vi "Sample_Scan_Pause_v2.vi"(4 "Z tilt comp":bool, 6 "Microsteps (MS=64)":dbl=64.0, 7 "Tilt x/z":dbl=64.0, 8 "Spacing [microns]":dbl=10.0, 9 "Long Side Speed [micron/s]":dbl=10.0, 10 "Scan Mode":T2 items=["Mode 1", "Mode 2", "Continuous 1", "Continuous 2"], 11 "waypoints path":path=path "C:/Users/ALS Measurement/Google Drive/LabVIEW/Thermionics Manipulator") -> (0 "velocity cluster":T1, 1 "Scan Time (hous:minutes:seconds)":string, 2 "Sample Scan Array":i32[][](array[numeric]), 3 "Problem":bool, 5 "Number of Points":i32)   [LabVIEW 2018]
uses:
  Scan Mode.ctl
  ConversionAndInformation/Unit_Control.ctl
panel:
  out "delta long side M3/1":dbl
  out "delta long side M2":dbl
  out "delta spacing M1/3":dbl
  out "delta spacing M2":dbl
  out "x/y":dbl
  out "in plain angle":dbl
  in  "velocity cluster 2":T1
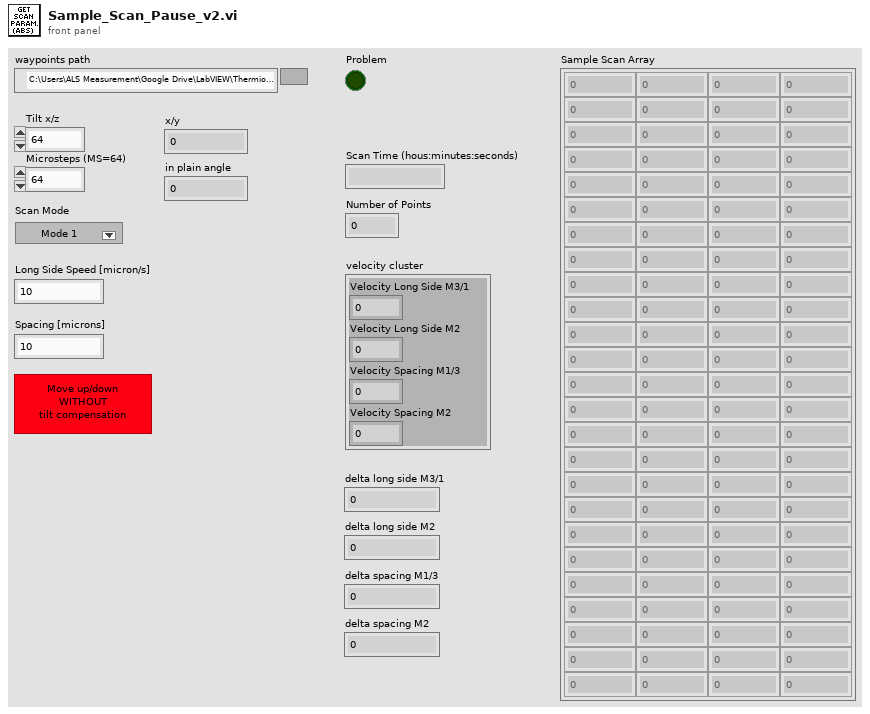
[diagram p1: front panel]
types:
  T1 = cluster{"Velocity Long Side M3/1":dbl, "Velocity Long Side M2":dbl, "Velocity Spacing M1/3":dbl, "Velocity Spacing M2":dbl}
  T2 = typedef "Scan Mode.ctl" = u16
  T3 = typedef "Unit_Control.ctl" = enum16{"Angle (Degrees)", "Rad", "Angle [TMC]", "Microsteps [TMC]", "Inches", "Nanometer", "Meter", "Centimeter", "Millimeter", "Micron"}
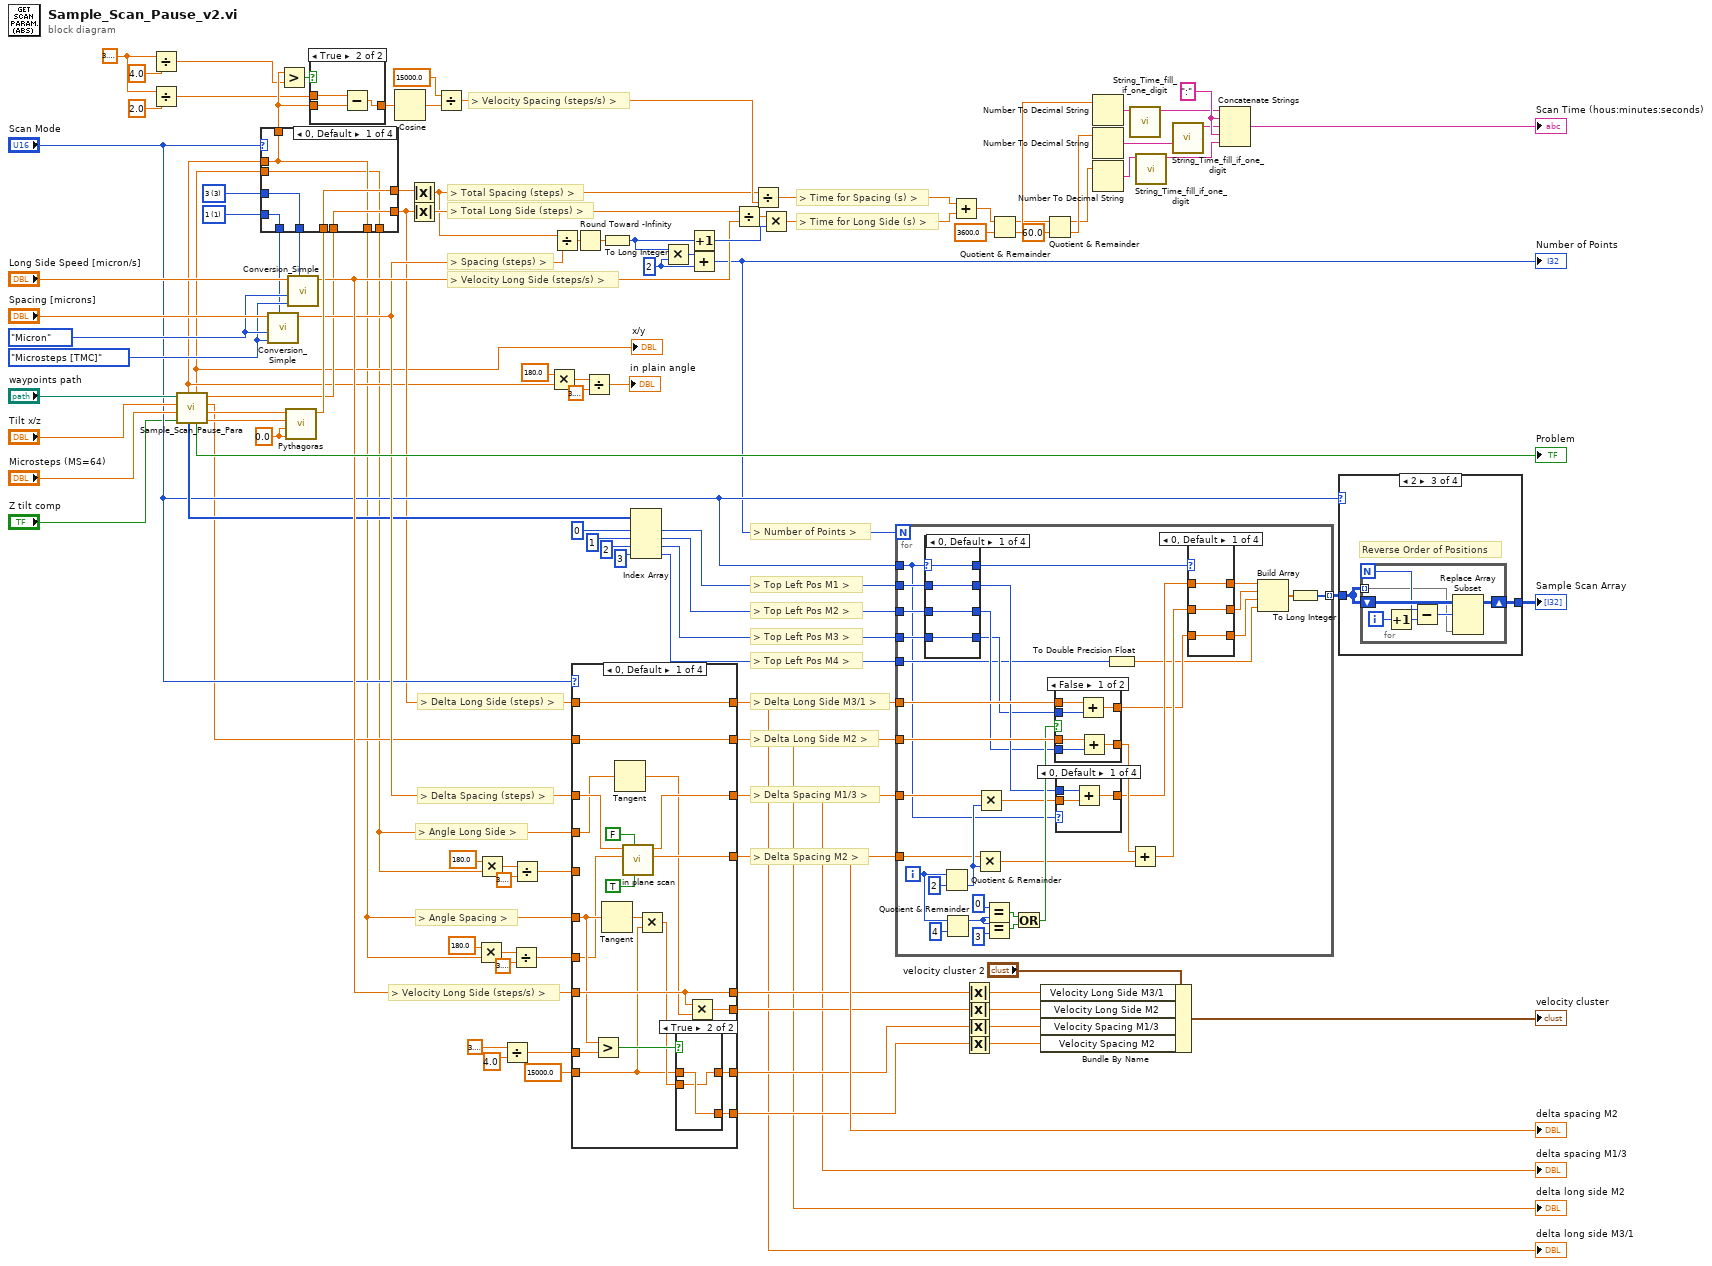
[diagram p0: block diagram]
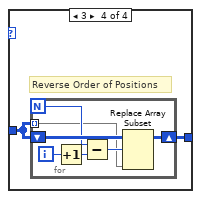
[diagram p4: hidden frame]
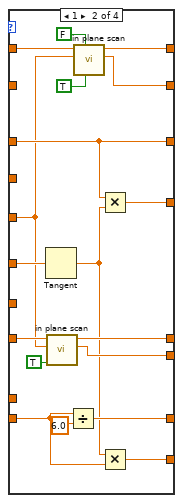
[diagram p6: hidden frame]
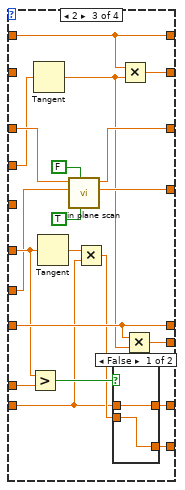
[diagram p7: hidden frame]
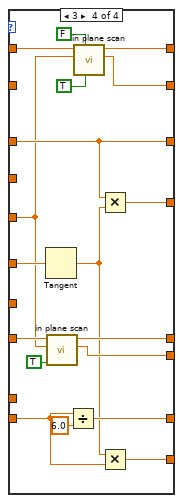
[diagram p9: hidden frame]
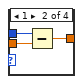
[diagram p10: hidden frame]
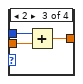
[diagram p11: hidden frame]
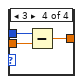
[diagram p12: hidden frame]
diagram:
  w54 = 3.141592653589793
  w79 = u16 3 items=["none", "1", "2", "3", "4", "all"] ("Motor")
  w80 = u16 1 items=["none", "1", "2", "3", "4", "all"] ("Motor")
  w83 = 2 ("y")
  w92 = ":"
  w101 = 0.0 ("Motor 2 Coordinate (bottom right)")
  w66 = Unit_Control."Microsteps [TMC]" ("Output Unit")
  w67 = Unit_Control."Micron" ("Input Unit")
  # "> Velocity Long Side (steps/s) >"
  # "> Top Left Pos M4 >"
  # "> Delta Spacing M2 >"
  # "> Delta Spacing M1/3 >"
  # "> Delta Long Side M2 >"
  # "> Delta Long Side M3/1 >"
  # "> Delta Spacing (steps) >"
  # "> Angle Spacing >"
  # "> Angle Long Side >"
  # "> Number of Points >"
  # "> Delta Long Side (steps) >"
  # "> Top Left Pos M3 >"
  # "> Top Left Pos M2 >"
  # "> Top Left Pos M1 >"
  # "> Time for Long Side (s) >"
  # "> Time for Spacing (s) >"
  # "> Total Long Side (steps) >"
  # "> Total Spacing (steps) >"
  # "> Velocity Spacing (steps/s) >"
  # "> Spacing (steps) >"
  # "> Velocity Long Side (steps/s) >"
  n1 = Divide(x=w54, y=4.0) -> (x/y=w53:dbl)
  n2 = Divide(x=w54, y=2.0) -> (x/y=w52:dbl)
  n3 = call "Sample_Scan_Pause_Para.vi"("Z tilt comp"="Z tilt comp", "Microsteps (MS=64)"="Microsteps (MS=64)", "Tilt x/z"="Tilt x/z", "waypoints path"="waypoints path") -> ("Delta M2 in plain total"=w102:dbl, "Delta M1 in plain total"=w103:dbl, "M2 Z tilt comp total"=w36:dbl, "Delta M3 total"=w35:dbl, "Problem"=→"Problem":bool, "tilt angle (rad)"=w19:dbl, "Top Left Position Array"=w49:i32[], "in plain angle (rad)"=w20:dbl)
  "x/y" <- w19
  n4 = call "Pythagoras.vi"("Motor 2 Coordinate (bottom right)"=w101, "Motor 1 Coordinate (bottom right)"=w101, "Motor 2 Coordinate (top left)"=w102, "Motor 1 Coordinate (top left)"=w103) -> ("In Plain Distance"=w65:dbl)  [unwired: 7 in]
  n5 = case shown="0, Default" "Scan Mode" {
    tunnel: w65 -> [w110 w119 w122 w131]
    tunnel: w35 -> [w113 w116 w125 w128]
    tunnel: [w113 w119 w125 w131] -> w34
    tunnel: [w112 w118 w124 w130] -> w64
    tunnel: [w111 w117 w123 w129] -> w81
    tunnel: w80 -> [w112 w117 w124 w129]
    tunnel: w79 -> [w111 w118 w123 w130]
    tunnel: [w110 w116 w122 w128] -> w5
    tunnel: w20 -> [w109 w114 w121 w126]
    tunnel: w19 -> [w108 w115 w120 w127]
    tunnel: [w109 w115 w121 w127] -> w72
    tunnel: [w109 w115 w121 w127] -> w9
    tunnel: [w108 w114 w120 w126] -> w12
    frame 0, Default {
    }
    frame 1 {
    }
    frame 2 {
    }
    frame 3 {
    }
  }
  n6 = call "Conversion_Simple.vi"("Motor"=w64, "Output Unit"=w66, "Input Unit"=w67, "Input"="Spacing [microns]") -> ("Output"=w57:dbl)  [unwired: 6 in, 1 out]
  n7 = Greater?(x=w72, y=w53) -> (0:w73:bool)
  n8 = call "Conversion_Simple.vi"("Motor"=w81, "Output Unit"=w66, "Input Unit"=w67, "Input"="Long Side Speed [micron/s]") -> ("Output"=w58:dbl)  [unwired: 6 in, 1 out]
  n9 = case shown="True" w73 {
    tunnel: w72 -> [w132 w135]
    tunnel: [w132 w134] -> w51
    tunnel: w52 -> [_ w133]
    frame False {
    }
    frame True {
      n10 = Subtract(x=w133, y=w135) -> (x-y=w134:dbl)
    }
  }
  n11 = Cosine(x=w51) -> (cos(x)=w71:dbl)
  n12 = Absolute Value(x=w5) -> (abs(x)=w4:dbl)
  n13 = Absolute Value(x=w34) -> (abs(x)=w33:dbl)
  n14 = Divide(x=15000.0, y=w71) -> (x/y=w70:dbl)
  n15 = Multiply(x=180.0 ("y"), y=w9) -> (x*y=w10:dbl)
  n16 = Multiply(x=180.0 ("y"), y=w12) -> (x*y=w15:dbl)
  n17 = Divide(x=3.141592653589793, y=4.0) -> (x/y=w38:dbl)
  n18 = Divide(x=w10, y=3.141592653589793) -> (x/y=w6:dbl)
  n19 = Divide(x=w15, y=3.141592653589793) -> (x/y=w7:dbl)
  n20 = Multiply(x=180.0 ("y"), y=w20) -> (x*y=w22:dbl)
  n21 = Divide(x=w4, y=w57) -> (x/y=w100:dbl)
  n22 = case shown="0, Default" "Scan Mode" {
    tunnel: w34 -> [w153 w175 w195 w217]
    tunnel: w9 -> [w140 w161 w181 w203]
    tunnel: w12 -> [w139 _ w180 _]
    tunnel: w57 -> [w152 w172 w194 w214]
    tunnel: [w153 w174 w195 w216] -> w16
    tunnel: [w137 w173 w191 w215] -> w17
    tunnel: [w151 w172 w193 w214] -> w18
    tunnel: [w150 w171 w192 w213] -> w63
    tunnel: w58 -> [w149 w170 w190 w212]
    tunnel: 15000.0 -> [w141 w163 w182 w205]
    tunnel: [w149 w168 w190 w210] -> w32
    tunnel: [w147 w167 w188 w209] -> w30
    tunnel: [w145 w166 w186 w208] -> w28
    tunnel: [w144 w164 w185 w206] -> w26
    tunnel: w38 -> [w138 _ w179 _]
    tunnel: w36 -> [w137 _ _ _]
    tunnel: w7 -> [_ w160 _ w202]
    tunnel: w6 -> [w136 _ w178 _]
    frame 0, Default {
      n23 = Greater?(x=w140, y=w138) -> (0:w146:bool)
      n24 = Tangent(1:w140) -> (0:w142:dbl)
      n25 = Tangent(1:w139) -> (0:w148:dbl)
      n26 = call "in plane scan.vi"("invert y"=TRUE, "invert x"=FALSE, "angle (degrees)"=w136, "v total"=w152) -> ("v_y"=w150:dbl, "v_x"=w151:dbl)  [unwired: 2 in, 4 out]
      n27 = Multiply(x=w142, y=w141) -> (x*y=w143:dbl)
      n28 = case shown="True" w146 {
        tunnel: w141 -> [w157 w159]
        tunnel: [w157 w158] -> w145
        tunnel: [w156 w159] -> w144
        tunnel: w143 -> [w156 w158]
        frame False {
        }
        frame True {
        }
      }
      n29 = Multiply(x=w149, y=w148) -> (x*y=w147:dbl)
    }
    frame 1 {
      n30 = Tangent(1:w161) -> (0:w162:dbl)
      n31 = call "in plane scan.vi"("abs(x,y)"=TRUE ("invert y"), "angle (degrees)"=w160, "v total"=w170) -> ("v_y"=w167:dbl, "v_x"=w168:dbl)  [unwired: 3 in, 4 out]
      n32 = Divide(x=w163, y=6.0) -> (x/y=w166:dbl)
      n33 = call "in plane scan.vi"("invert y"=TRUE, "invert x"=FALSE, "angle (degrees)"=w160, "v total"=w175) -> ("v_y"=w173:dbl, "v_x"=w174:dbl)  [unwired: 2 in, 4 out]
      n34 = Multiply(x=w172, y=w162) -> (x*y=w171:dbl)
      n35 = Multiply(x=w162, y=w163) -> (x*y=w164:dbl)
    }
    frame 2 {
      n36 = Greater?(x=w181, y=w179) -> (0:w187:bool)
      n37 = Tangent(1:w180) -> (0:w189:dbl)
      n38 = Tangent(1:w181) -> (0:w183:dbl)
      n39 = call "in plane scan.vi"("invert y"=TRUE, "invert x"=FALSE, "angle (degrees)"=w178, "v total"=w194) -> ("v_y"=w192:dbl, "v_x"=w193:dbl)  [unwired: 2 in, 4 out]
      n40 = Multiply(x=w183, y=w182) -> (x*y=w184:dbl)
      n41 = case shown="False" w187 {
        tunnel: w182 -> [w199 w201]
        tunnel: [w199 w200] -> w186
        tunnel: [w198 w201] -> w185
        tunnel: w184 -> [w198 w200]
        frame False {
        }
        frame True {
        }
      }
      n42 = Multiply(x=w195, y=w189) -> (x*y=w191:dbl)
      n43 = Multiply(x=w190, y=w189) -> (x*y=w188:dbl)
    }
    frame 3 {
      n44 = Tangent(1:w203) -> (0:w204:dbl)
      n45 = call "in plane scan.vi"("abs(x,y)"=TRUE ("invert y"), "angle (degrees)"=w202, "v total"=w212) -> ("v_y"=w209:dbl, "v_x"=w210:dbl)  [unwired: 3 in, 4 out]
      n46 = Divide(x=w205, y=6.0) -> (x/y=w208:dbl)
      n47 = call "in plane scan.vi"("invert y"=TRUE, "invert x"=FALSE, "angle (degrees)"=w202, "v total"=w217) -> ("v_y"=w215:dbl, "v_x"=w216:dbl)  [unwired: 2 in, 4 out]
      n48 = Multiply(x=w214, y=w204) -> (x*y=w213:dbl)
      n49 = Multiply(x=w204, y=w205) -> (x*y=w206:dbl)
    }
  }
  "delta spacing M2" <- w63
  "delta spacing M1/3" <- w18
  "delta long side M2" <- w17
  "delta long side M3/1" <- w16
  n50 = Round Toward -Infinity(1:w100) -> (0:w99:dbl)
  n51 = Divide(x=w22, y=3.141592653589793) -> (x/y=→"in plain angle":dbl)
  n52 = To Long Integer(number=w99) -> (32bit integer=w82:i32)
  n53 = Index Array(array=w49, index #1=0 ("index"), index #2=1 ("index"), index #3=2 ("index"), index #4=3 ("index")) -> (element #1=w44:i32, element #2=w43:i32, element #3=w42:i32, element #4=w41:i32)
  n54 = Multiply(x=w82, y=w83) -> (x*y=w84:i32)
  n55 = Increment(x=w82) -> (x+1=w77:i32)
  n56 = Add(x=w84, y=w83) -> (x+y=w2:i32)
  "Number of Points" <- w2
  n57 = Divide(x=w33, y=w58) -> (x/y=w78:dbl)
  n58 = Divide(x=w4, y=w70) -> (x/y=w75:dbl)
  n59 = Multiply(x=w78, y=w77) -> (x*y=w76:dbl)
  n60 = for {
    N: w2 -> [_]
    tunnel: w44 -> [w237]
    tunnel: w43 -> [w236]
    tunnel: w42 -> [w233]
    tunnel: [w221] -> w62 mode=indexing
    tunnel: w41 -> [w224]
    tunnel: w16 -> [w243]
    tunnel: w17 -> [w242]
    tunnel: w18 -> [w245]
    tunnel: w63 -> [w244]
    tunnel: "Scan Mode" -> [w220]
    i -> [w252]
    n61 = case shown="0, Default" w220 {
      selector: w220 -> [w279 w283 w287 w291]
      tunnel: w237 -> [w282 w284 w290 w292]
      tunnel: w236 -> [w281 w285 w289 w293]
      tunnel: w233 -> [w280 w286 w288 w294]
      tunnel: [w282 w286 w290 w294] -> w235
      tunnel: [w281 w285 w289 w293] -> w234
      tunnel: [w280 w284 w288 w292] -> w232
      tunnel: [w279 w283 w287 w291] -> w231
      frame 0, Default {
      }
      frame 1 {
      }
      frame 2 {
      }
      frame 3 {
      }
    }
    n62 = Quotient & Remainder(x=w252, y=2) -> (floor(x/y)=w246:i32)  [unwired: 1 out]
    n63 = Quotient & Remainder(x=w252, y=4) -> (x-y*floor(x/y)=w247:i32)  [unwired: 1 out]
    n64 = Multiply(x=w244, y=w246) -> (x*y=w240:dbl)
    n65 = Multiply(x=w245, y=w246) -> (x*y=w239:dbl)
    n66 = Equal?(x=0 ("y"), y=w247) -> (x = y?=w249:bool)
    n67 = Equal?(x=w247, y=3) -> (x = y?=w248:bool)
    n68 = Or(x=w249, y=w248) -> (x .or. y?=w241:bool)
    n69 = case shown="False" w241 {
      tunnel: w242 -> [w299 _]
      tunnel: w243 -> [w300 _]
      tunnel: w234 -> [w298 w301]
      tunnel: w232 -> [w297 w302]
      tunnel: [w296 w302] -> w228
      tunnel: [w295 w301] -> w238
      frame False {
        n70 = Add(x=w300, y=w297) -> (x+y=w296:dbl)
        n71 = Add(x=w299, y=w298) -> (x+y=w295:dbl)
      }
      frame True {
      }
    }
    n72 = case shown="0, Default" w220 {
      tunnel: w239 -> [w257 w260 w263 w266]
      tunnel: w235 -> [w256 w259 w262 w265]
      tunnel: [w255 w258 w261 w264] -> w230
      frame 0, Default {
        n73 = Add(x=w256, y=w257) -> (x+y=w255:dbl)
      }
      frame 1 {
        n74 = Subtract(x=w259, y=w260) -> (x-y=w258:dbl)
      }
      frame 2 {
        n75 = Add(x=w262, y=w263) -> (x+y=w261:dbl)
      }
      frame 3 {
        n76 = Subtract(x=w265, y=w266) -> (x-y=w264:dbl)
      }
    }
    n77 = To Double Precision Float(number=w224) -> (double precision float=w223:dbl)
    n78 = Add(x=w238, y=w240) -> (x+y=w229:dbl)
    n79 = case shown="0, Default" w231 {
      tunnel: w230 -> [w269 w270 w275 w276]
      tunnel: w229 -> [w268 w271 w274 w277]
      tunnel: w228 -> [w267 w272 w273 w278]
      tunnel: [w269 w272 w275 w278] -> w227
      tunnel: [w268 w271 w274 w277] -> w226
      tunnel: [w267 w270 w273 w276] -> w225
      frame 0, Default {
      }
      frame 1 {
      }
      frame 2 {
      }
      frame 3 {
      }
    }
    n80 = Build Array(w227, w226, w225, w223) -> (w222:dbl[])
    n81 = To Long Integer(number=w222) -> (32bit integer=w221:i32[])
  }
  n82 = Add(x=w75, y=w76) -> (x+y=w74:dbl)
  n83 = Absolute Value(x=w32) -> (abs(x)=w31:dbl)
  n84 = Absolute Value(x=w30) -> (abs(x)=w29:dbl)
  n85 = Absolute Value(x=w28) -> (abs(x)=w27:dbl)
  n86 = Absolute Value(x=w26) -> (abs(x)=w25:dbl)
  n87 = Quotient & Remainder(x=w74, y=3600.0) -> (x-y*floor(x/y)=w95:dbl, floor(x/y)=w97:dbl)
  n88 = Bundle By Name(cluster="velocity cluster 2", "Velocity Long Side M3/1"=w31, "Velocity Long Side M2"=w29, "Velocity Spacing M1/3"=w27, "Velocity Spacing M2"=w25) -> (→"velocity cluster":T1)
  n89 = Quotient & Remainder(x=w95, y=60.0) -> (x-y*floor(x/y)=w93:dbl, floor(x/y)=w94:dbl)
  n90 = Number To Decimal String(number=w97) -> (decimal integer string=w90:string)  [unwired: 1 in]
  n91 = Number To Decimal String(number=w94) -> (decimal integer string=w88:string)  [unwired: 1 in]
  n92 = Number To Decimal String(number=w93) -> (decimal integer string=w86:string)  [unwired: 1 in]
  n93 = call "String_Time_fill_if_one_digit.vi"("String"=w90) -> ("String 2"=w89:string)  [unwired: 10 in]
  n94 = call "String_Time_fill_if_one_digit.vi"("String"=w86) -> ("String 2"=w85:string)  [unwired: 10 in]
  n95 = call "String_Time_fill_if_one_digit.vi"("String"=w88) -> ("String 2"=w87:string)  [unwired: 10 in]
  n96 = Concatenate Strings(w89, w92, w87, w92, w85) -> (→"Scan Time (hous:minutes:seconds)":string)
  n97 = case shown="2" "Scan Mode" {
    tunnel: w62 -> [w303 w304 w306 w315]
    tunnel: [w303 w304 w305 w314] -> w3
    frame 0, Default {
    }
    frame 1 {
    }
    frame 2 {
      # "Reverse Order of Positions"
      n98 = for {
        N -> [w311]
        tunnel: w306 -> [w309] mode=indexing
        shift-right: [w312] -> w305
        shift-left: w306 -> [w313]
        i -> [w308]
        n99 = Increment(x=w308) -> (x+1=w307:i32)
        n100 = Subtract(x=w311, y=w307) -> (x-y=w310:i32)
        n101 = Replace Array Subset(array=w313, new element=w309, index (row)=w310) -> (w312:i32[][])  [unwired: 1 in]
      }
    }
    frame 3 {
      # "Reverse Order of Positions"
      n102 = for {
        N -> [w320]
        tunnel: w315 -> [w318] mode=indexing
        shift-right: [w321] -> w314
        shift-left: w315 -> [w322]
        i -> [w317]
        n103 = Increment(x=w317) -> (x+1=w316:i32)
        n104 = Subtract(x=w320, y=w316) -> (x-y=w319:i32)
        n105 = Replace Array Subset(array=w322, new element=w318, index (row)=w319) -> (w321:i32[][])  [unwired: 1 in]
      }
    }
  }
  "Sample Scan Array" <- w3
